vi "Get DPD LUT String.vi"(8 "error in (no error)":errorcluster, 11 "Test Group In":refnum<data-value>) -> (0 "error out":errorcluster, 2 "DPD LUT":string, 3 "Test Group Out":refnum<data-value>)   [LabVIEW 2016, in "Test Group Manager.lvlib" / "Test Group.lvclass"]
uses:
  Test Group.lvclass
  Test Group.lvclass/Test Group.ctl
  Read Input Power Initialized.vi
  Read Test Group Data.vi
  <vilib>/Utility/error.llb/Error Cluster From Error Code.vi
  <vilib>/ErrorRing/Error Ring.xnode
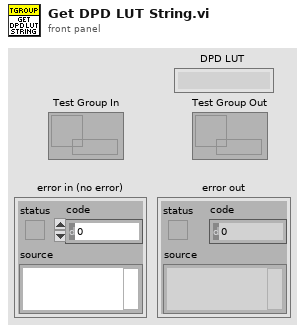
[diagram p1: front panel]
types:
  T1 = cluster{"DPD LUT Name":string, "Input Power":string}
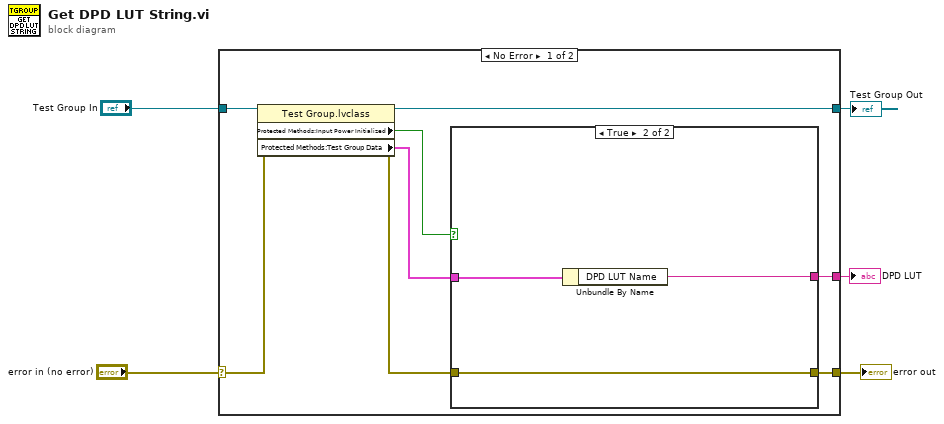
[diagram p0: block diagram]
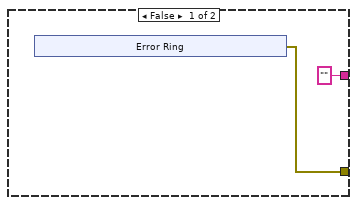
[diagram p2: hidden frame]
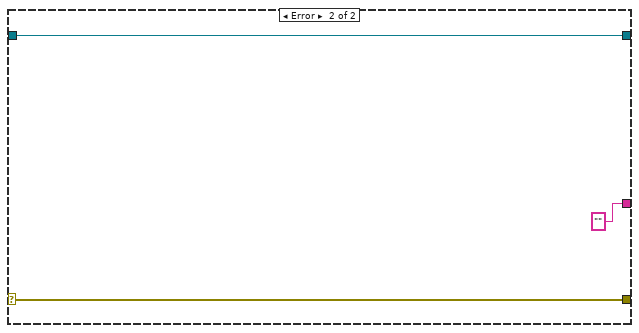
[diagram p3: hidden frame]
diagram:
  n1 = case shown="No Error" "error in (no error)" {
    selector: "error in (no error)" -> [w13 w26]
    tunnel: [w9 w26] -> w4
    tunnel: [w11 w25] -> w1
    tunnel: "Test Group In" -> [w12 w25]
    tunnel: [w6 "" ("Input Power 2")] -> w3
    frame No Error {
      n2 = property class="Test Group.lvclass"(reference=w12, error in=w13) -> (reference out=w11:refnum<data-value>, error out=w8:errorcluster, "Protected Methods:Input Power Initialized"=w10:bool, "Protected Methods:Test Group Data"=w7:T1)
      n3 = case shown="True" w10 {
        tunnel: [w15 w23] -> w9
        tunnel: w8 -> [_ w23]
        tunnel: w7 -> [_ w22]
        tunnel: ["" ("Input Power") w21] -> w6
        frame False {
          n4 = xnode "Error Ring"() -> ("error out"=w15:errorcluster)
        }
        frame True {
          n5 = Unbundle By Name(w22) -> ("DPD LUT Name"=w21:string)
        }
      }
    }
    frame Error {
    }
  }
  "error out" <- w4
  "DPD LUT" <- w3
  "Test Group Out" <- w1
